vi "FPGA Main 7-7 (Container).vi"   [LabVIEW 2017]
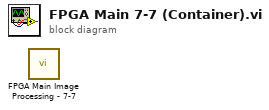
[diagram p0: block diagram]
diagram:
  n1 = call "FPGA Main Image Processing - 7-7.vi"() -> ()  [unwired: 12 in]
